vi "Actor Core.vi"(8 "Error In":errorcluster, 11 "CS++SeqEditor in":refnum<class "CS++SeqEditor.lvclass">) -> (0 "Error Out":errorcluster, 3 "Actor out":refnum<class "Actor.lvclass">)   [LabVIEW 2016, in "CS++SeqEditor.lvlib" / "CS++SeqEditor.lvclass"]
doc: "(<B>Filename</B>: Actor Framework.lvlib:Actor.lvclass:Actor Core.vi)\n\nReceives messages to the actor, reacts to them, and initiates any error handling that may shut the actor down.\n\nDescendant classes may override this VI to append parallel tasks for the actor to complete while it handles messages. Overrides use the Call Parent Method node."
uses:
  CS++SeqEditor.lvclass
  C:/User/Brand/LVP/CSPP-Dev/Packages/CSPP_Core/Actors/CS++BaseActor/CS++BaseActor.lvclass
  C:/User/Brand/LVP/CSPP-Dev/Packages/CSPP_Core/Actors/CS++GUIActor/CS++GUIActor.lvclass
  C:/Program Files (x86)/National Instruments/LabVIEW 2016/vi.lib/ActorFramework/Actor/Actor.lvclass
  <vilib>/ActorFramework/Actor/Actor.lvclass
  CSPP_Core/Libraries/Base/FGV Action.ctl
  CSPP_Core/Actors/CS++BaseActor/CS++BaseActor.lvclass/CS++BaseActor.ctl
  CSPP_Core/Actors/CS++GUIActor/CS++GUIActor.lvclass/CS++GUIActor.ctl
  CS++SeqEditor.lvclass/CS++SeqEditor.ctl
  <vilib>/ActorFramework/Actor/Actor.lvclass/Actor.ctl
  <vilib>/ActorFramework/Message Enqueuer/Message Enqueuer.lvclass/Message Enqueuer.ctl
  CS++SeqEditor Messages/Load Sequence Msg/Load Sequence Msg.lvclass/Load Sequence Msg.ctl
  CS++SeqEditor Messages/Save Sequence Msg/Save Sequence Msg.lvclass/Save Sequence Msg.ctl
  <vilib>/ActorFramework/Message/Message.lvclass
  CSPP_Core/Actors/CS++BaseActor/Read Object Name.vi
  CSPP_Core/Actors/CS++GUIActor/Read Associated Actor Name.vi
  CSPP_Core/Actors/CS++GUIActor/Read Stop-Event.vi
  CSPP_Core/Actors/CS++GUIActor/Read PV-Update.vi
  <vilib>/ActorFramework/Message Enqueuer/Init from Existing Queue.vi
  <vilib>/ActorFramework/Message Enqueuer/Enqueue.vi
  <vilib>/ActorFramework/Stop Msg/Stop Msg.lvclass
  C:/Program Files (x86)/National Instruments/LabVIEW 2016/vi.lib/ActorFramework/Message/Message.lvclass
  CS++SeqEditor Messages/Load Sequence Msg/Load Sequence Msg.lvclass
  CS++SeqEditor Messages/Save Sequence Msg/Save Sequence Msg.lvclass
  <vilib>/ActorFramework/Message Priority Queue/Priority Enqueue.vi
  CSPP_Core/Classes/CS++BaseClasses/Factory/CS++Factory.lvclass
  CSPP_Core/Classes/CS++ProcessVariables/ProcessVariable/PV.lvclass
  <vilib>/ActorFramework/Message Enqueuer/Message Enqueuer.lvclass
  CSPP_Core/Actors/CS++GUIActor/CS++GUIActor.lvclass
  CSPP_Core/Actors/CS++BaseActor/CS++BaseActor.lvclass
  CSPP_Core/Libraries/Base/CS++Base.lvlib
  CSPP_Core/Libraries/Utilities/CS++Utilities.lvlib
panel:
  out "Drop String":string
  in  "Message Tree":string(tree)
  out "Selected Path":path
  in  "Stop Button":bool
  out "Associated DeviceActor":string
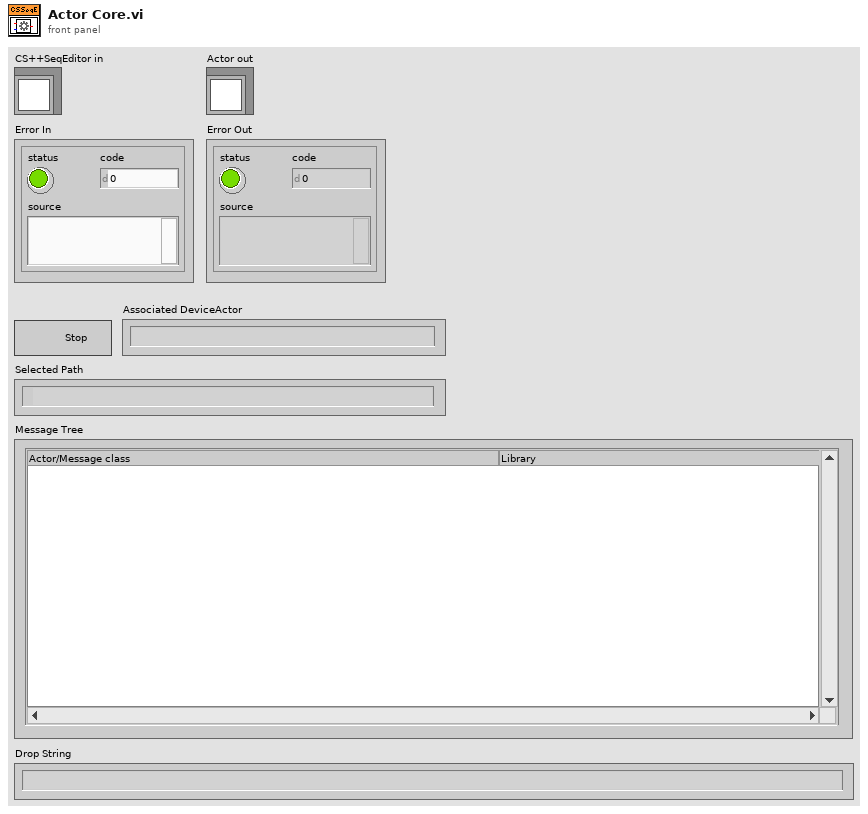
[diagram p1: front panel]
types:
  T1 = typedef "CS++Base.lvlib/FGV Action.ctl" = enum16{"add", "replace", "read", "remove", "reset", "get attributes"}
  T2 = enum32{"Invalid", "Standard", "Closed", "Hidden", "Minimized", "Maximized"}
  T3 = cluster{"Navigate Tree:Get Path":string[], "Actor Framework:Message":refnum<class "Message.lvclass">}
  T4 = typedef "LVMenuShortCut.ctl" = cluster{"include Shift key?":bool, "include Ctrl key?":bool, "shortcut key":string}
  T5 = cluster{"data name":string, "drag data":variant}[]
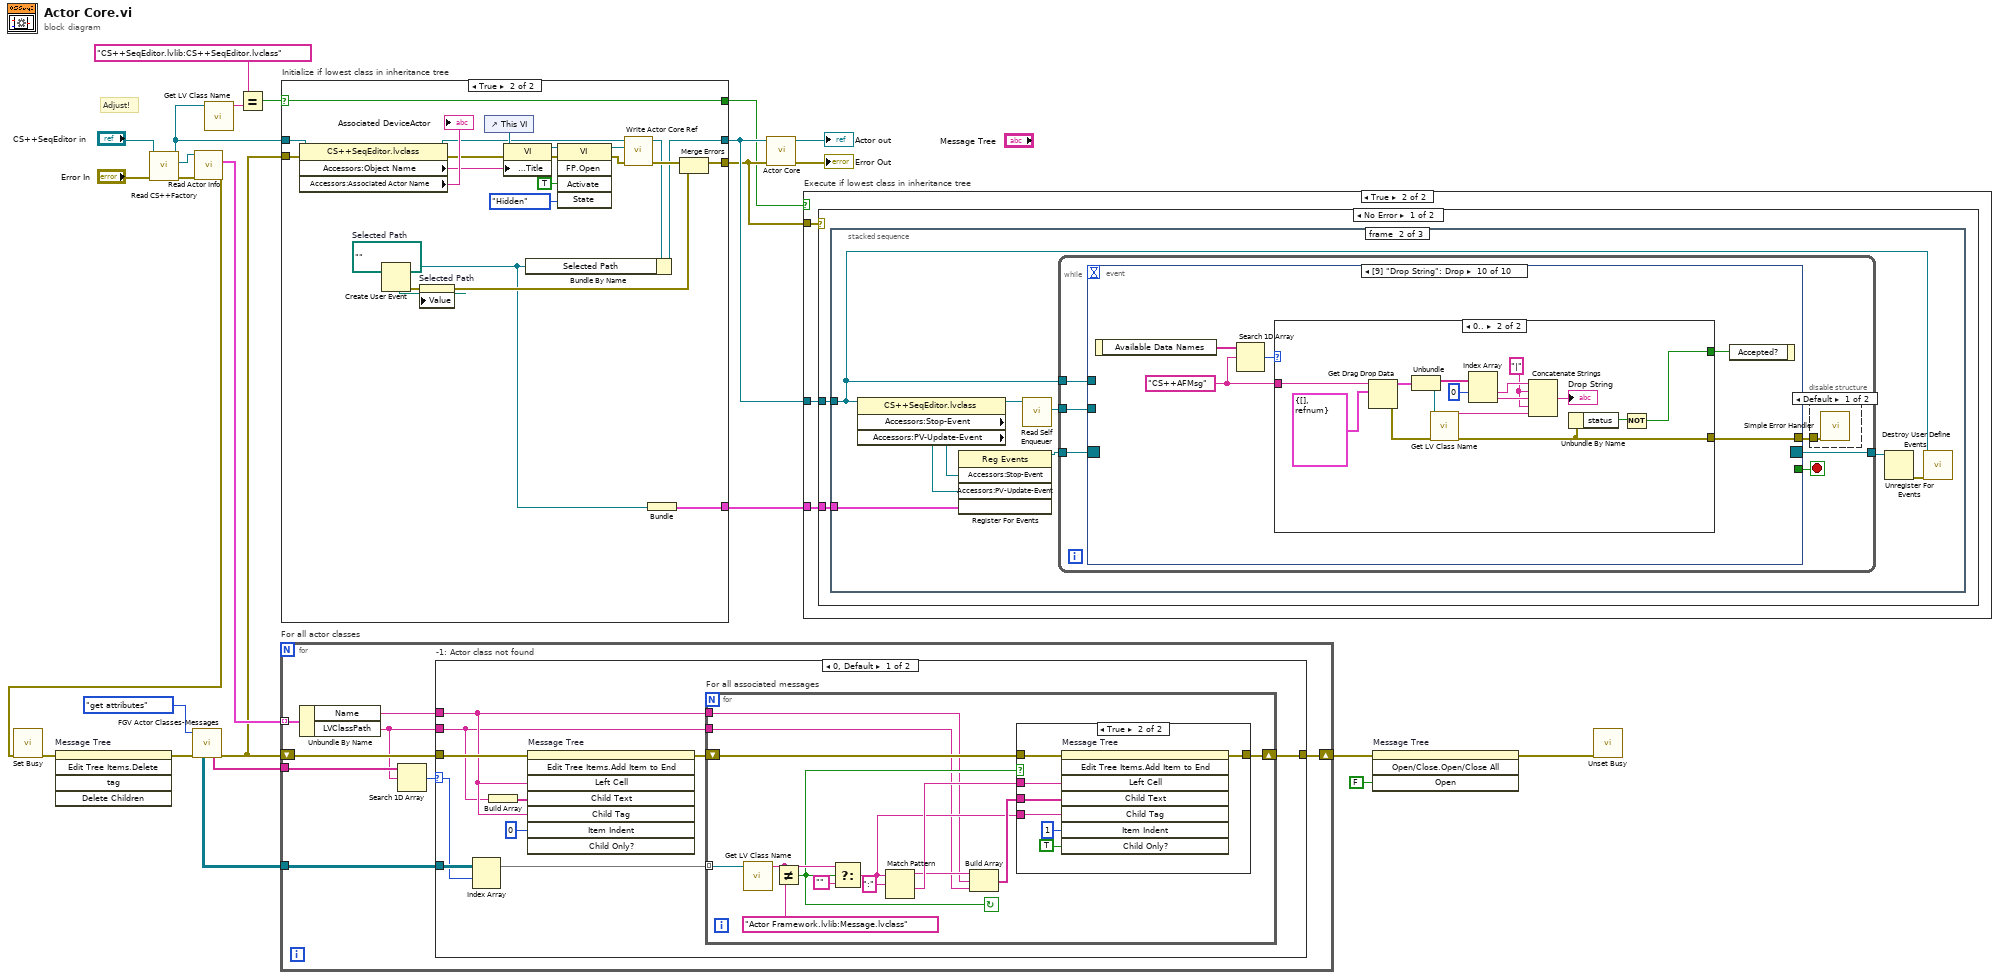
[diagram p0: block diagram]
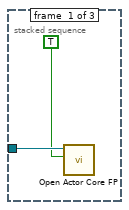
[diagram p5: hidden frame]
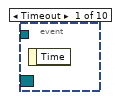
[diagram p6: hidden frame]
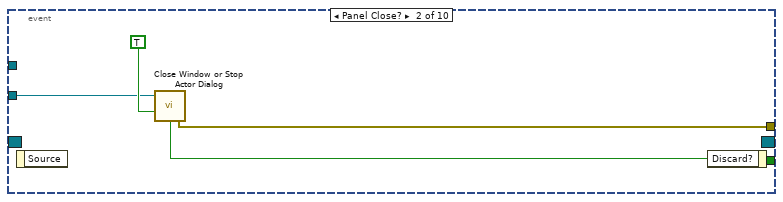
[diagram p7: hidden frame]
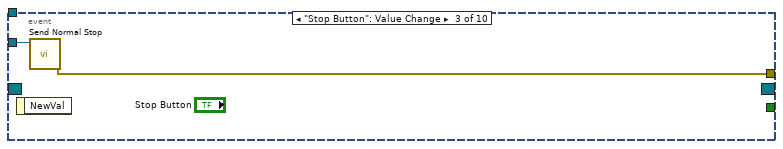
[diagram p8: hidden frame]
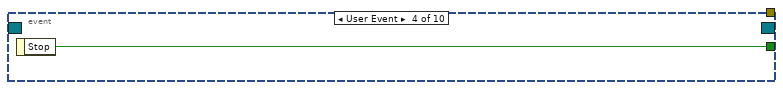
[diagram p9: hidden frame]
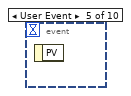
[diagram p10: hidden frame]
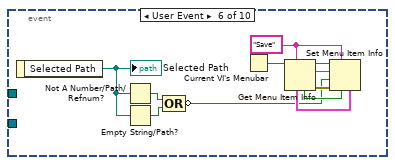
[diagram p11: hidden frame]
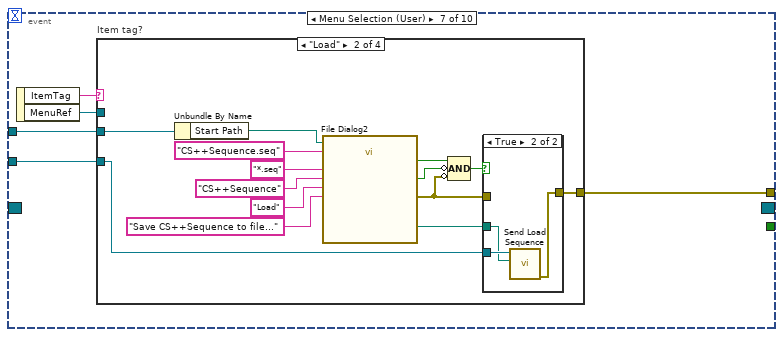
[diagram p12: hidden frame]
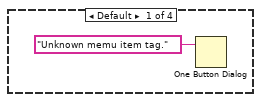
[diagram p13: hidden frame]
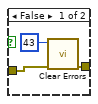
[diagram p14: hidden frame]
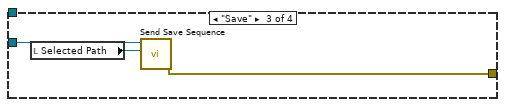
[diagram p15: hidden frame]
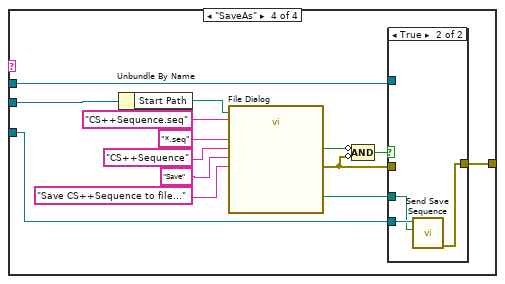
[diagram p16: hidden frame]
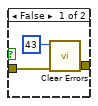
[diagram p17: hidden frame]
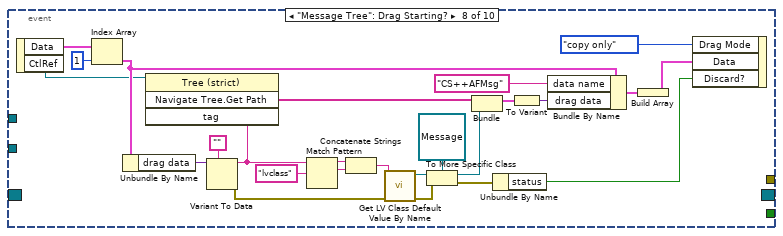
[diagram p18: hidden frame]
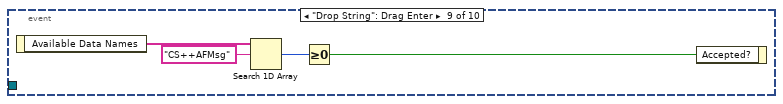
[diagram p19: hidden frame]
diagram:
  # "Adjust!"
  n1 = call "Read CS++Factory.vi"("error in (no error)"="Error In", "CS++BaseActor in"="CS++SeqEditor in") -> ("error out"=w7:errorcluster, "CS++Factory"=w8:refnum<class "CS++Factory.lvclass">, "CS++BaseActor out"=w4:refnum<class "CS++SeqEditor.lvclass">)  [unwired: 7 in]
  n2 = call-dynamic "Read Actor Info.vi"("Error In"=w7, "CS++Factory in"=w8) -> ("Error Out"=w2:errorcluster, "Actors"=w3:cluster{"Name":string, "LVClassPath":string}[])  [unwired: 7 in, 1 out]
  n3 = call <vilib>:"Set Busy.vi"("error in (no error)"=w2) -> ("error out"=w10:errorcluster)  [unwired: 9 in, 1 out]
  n4 = invoke on="Message Tree" class="Tree (strict)" method="Edit Tree Items.Delete"(error in=w10) -> (error out=w11:errorcluster)  [unwired: 4 in, 4 out]
  n5 = call "FGV Actor Classes-Messages.vi"("Error In"=w11, "Action (read)"=FGV_Action."get attributes") -> ("Error Out"=w1:errorcluster, "Class Names"=w14:string[], "CS++Messages"=w15:refnum<class "Message.lvclass">[][])  [unwired: 5 in, 2 out]
  n6 = call <vilib>:"Get LV Class Name.vi"("object"=w4) -> ("class name"=w25:string)  [unwired: 9 in, 1 out]
  n7 = Equal?(x="CS++SeqEditor.lvlib:CS++SeqEditor.lvclass" ("class name"), y=w25) -> (x = y?=w21:bool)
  n8 = for "For all actor classes" {
    tunnel: w15 -> [w33]
    tunnel: w14 -> [w28]
    shift-right: [w31] -> w12
    shift-left: w1 -> [w32]
    tunnel: w3 -> [w30] mode=indexing
    n9 = Unbundle By Name(w30) -> ("Name"=w29:string, "LVClassPath"=w27:string)
    n10 = Search 1D Array(1D array=w28, element=w27) -> (index of element=w26:i32)  [unwired: 1 in]
    n11 = case "-1: Actor class not found" shown="0, Default" w26 {
      selector: w26 -> [w36 _]
      tunnel: w33 -> [w43 _]
      tunnel: w32 -> [w42 w66]
      tunnel: [w39 w66] -> w31
      tunnel: w29 -> [w35 _]
      tunnel: w27 -> [w34 _]
      frame 0, Default {
        n12 = Index Array(array=w43, index (row)=w36) -> (element=w37:refnum<class "Message.lvclass">[])  [unwired: 1 in]
        n13 = Build Array(w34) -> (w38:string[])
        n14 = invoke on="Message Tree" class="Tree (strict)" method="Edit Tree Items.Add Item to End"(error in=w42, "Left Cell"=w35, "Child Text"=w38, "Child Tag"=w35, "Item Indent"=0 ("New Item Indentation")) -> (error out=w40:errorcluster)  [unwired: 3 in, 7 out]
        n15 = for "For all associated messages" {
          tunnel: w37 -> [w57] mode=indexing
          shift-right: [w51] -> w39
          shift-left: w40 -> [w52]
          tunnel: w35 -> [w45]
          tunnel: w34 -> [w44]
          stop <- w46 continue-if-true
          n16 = call <vilib>:"Get LV Class Name.vi"("object"=w57) -> ("class name"=w55:string)  [unwired: 9 in, 1 out]
          n17 = Not Equal?(x=w55, y="Actor Framework.lvlib:Message.lvclass") -> (x != y?=w46:bool)
          n18 = Select(t=w55, s=w46, f="") -> (s? t:f=w47:string)
          n19 = Match Pattern(string=w47, regular expression=":") -> (before substring=w49:string, after substring=w50:string)  [unwired: 1 in, 2 out]
          n20 = Build Array(w49, w45, w44) -> (w48:string[])
          n21 = case shown="True" w46 {
            tunnel: w52 -> [w58 w65]
            tunnel: [w58 w64] -> w51
            tunnel: w50 -> [_ w63]
            tunnel: w48 -> [_ w62]
            tunnel: w47 -> [_ w61]
            frame False {
            }
            frame True {
              n22 = invoke on="Message Tree" class="Tree (strict)" method="Edit Tree Items.Add Item to End"(error in=w65, "Left Cell"=w63, "Child Text"=w62, "Child Tag"=w61, "Item Indent"=1 ("New Item Indentation"), "Child Only?"=TRUE) -> (error out=w64:errorcluster)  [unwired: 2 in, 7 out]
            }
          }
        }
      }
      frame -1 {
      }
    }
  }
  n23 = case "Initialize if lowest class in inheritance tree" shown="True" w21 {
    selector: w21 -> [w69 w90]
    tunnel: w1 -> [w67 w87]
    tunnel: w4 -> [w68 w88]
    tunnel: [w68 w75] -> w23
    tunnel: [w67 w73] -> w22
    tunnel: [w69 w90] -> w20
    tunnel: [_ w70] -> w17
    frame False {
    }
    frame True {
      w77 = path ""  # Selected Path
      n24 = property class="CS++SeqEditor.lvclass"(reference=w88, error in=w87) -> (reference out=w78:refnum<class "CS++SeqEditor.lvclass">, error out=w80:errorcluster, "Accessors:Object Name"=w79:string, "Accessors:Associated Actor Name"=→"Associated DeviceActor":string)
      n25 = Create User Event(user event datatype=w77) -> (user event=w71:refnum<user-event>, error out=w74:errorcluster)  [unwired: 1 in]
      n26 = property on="Selected Path" class="Path"(error in=w74, "Value"=w77) -> (error out=w72:errorcluster)  [unwired: 1 in, 1 out]
      n27 = control-ref of="This VI"() -> (w83:refnum<vi>)
      n28 = property class="VI"(reference=w83, error in=w80, "Front Panel.Title"=w79) -> (reference out=w82:refnum<vi>, error out=w81:errorcluster)
      n29 = invoke class="VI" method="FP.Open"(reference=w82, error in=w81, "Activate"=TRUE ("Activate?"), "State"=T2."Hidden") -> (reference out=w89:refnum<vi>, error out=w85:errorcluster)  [unwired: 1 in, 3 out]
      n30 = call "Write Actor Core Ref.vi"("error in (no error)"=w85, "Actor Core Ref"=w89, "CS++BaseActor in"=w78) -> ("error out"=w84:errorcluster, "CS++BaseActor out"=w76:refnum<class "CS++SeqEditor.lvclass">)  [unwired: 7 in]
      n31 = Bundle By Name(cluster=w76, "Selected Path"=w71) -> (w75:refnum<class "CS++SeqEditor.lvclass">)
      n32 = Bundle("Selected Path"=w71) -> (w70:cluster{"Selected Path":refnum<user-event>})  [unwired: 1 in]
      n33 = Merge Errors(w84, w72) -> (w73:errorcluster)
    }
  }
  n34 = call-parent "Actor Core.vi"("error in"=w22, "CS++GUIActor in"=w23) -> ("error out"=→"Error Out":errorcluster, "Actor out"=→"Actor out":refnum<class "Actor.lvclass">)  [unwired: 8 in]
  n35 = case "Execute if lowest class in inheritance tree" shown="True" w20 {
    tunnel: w23 -> [_ w95]
    tunnel: w22 -> [_ w94]
    tunnel: w17 -> [_ w93]
    frame False {
    }
    frame True {
      n36 = case shown="No Error" w94 {
        tunnel: w95 -> [w97 _]
        tunnel: w93 -> [w96 _]
        frame No Error {
          n37 = stacked-sequence {
            tunnel: w97 -> [w99 w101 w232]
            tunnel: w96 -> [_ w100 _]
            frame #0 {
              n38 = call "Open Actor Core FP.vi"("Open FP (F)"=TRUE, "CS++BaseActor in"=w99) -> ()  [unwired: 8 in, 2 out]
            }
            frame #1 {
              n39 = property class="CS++SeqEditor.lvclass"(reference=w101) -> (reference out=w106:refnum<class "CS++SeqEditor.lvclass">, "Accessors:Stop-Event"=w103:refnum<user-event>, "Accessors:PV-Update-Event"=w102:refnum<user-event>)  [unwired: 1 in, 1 out]
              n40 = register-events(w103, w102, w100) -> (reference out=w104:refnum<event-registration>)  [unwired: 2 in, 1 out]
              n41 = call <vilib>:"Read Self Enqueuer.vi"("Actor"=w106) -> ("Self Enqueuer"=w105:refnum<class "Message Enqueuer.lvclass">)  [unwired: 10 in]
              n42 = while {
                tunnel: w104 -> [w114]
                tunnel: [w112] -> w108
                tunnel: w105 -> [w110]
                tunnel: w101 -> [w109]
                stop <- w113 stop-if-true
                n43 = event shown="[9] \"Drop String\": Drop" {
                  selector: w114 -> [_ _ _ _ _ _ _ _ _ _]
                  dyn-events: [_ _ _ _ _ _ _ _ _ _] -> w112
                  timeout: _ -> [_ _ _ _ _ _ _ _ _ _]
                  tunnel: [_ _ _ w120 _ _ _ _ _ _] -> w113
                  tunnel: [_ w115 w119 _ _ _ w132 _ _ w211] -> w111
                  tunnel: w110 -> [_ w116 w118 _ _ _ w133 _ _ _]
                  tunnel: w109 -> [_ _ _ _ _ _ w135 _ _ _]
                  event Timeout {
                    n44 = event-data() -> ()  [unwired: 1 in, 1 out]
                  }
                  event Panel Close? {
                    n45 = event-data() -> ()  [unwired: 1 in, 1 out]
                    n46 = call "Close Window or Stop Actor Dialog.vi"("Self Enqueuer"=w116) -> ("Error Out"=w115:errorcluster)  [unwired: 2 in]
                    n47 = event-data("Discard?"=TRUE) -> ()  [unwired: 1 in, 1 out]
                  }
                  event "Stop Button": Value Change {
                    n48 = event-data() -> ()  [unwired: 1 in, 1 out]
                    n49 = call <vilib>:"Send Normal Stop.vi"("Message Enqueuer"=w118) -> ("error out"=w119:errorcluster)  [unwired: 10 in]
                  }
                  event User Event {
                    n50 = event-data() -> ("Stop"=w120:bool)  [unwired: 1 in]
                  }
                  event User Event {
                    n51 = event-data() -> ()  [unwired: 1 in, 1 out]
                  }
                  event User Event {
                    w128 = "Save"
                    n52 = event-data() -> ("Selected Path"=w126:path)  [unwired: 1 in]
                    "Selected Path" <- w126
                    n53 = Not A Number/Path/Refnum?(number/path/refnum=w126) -> (NaN/Path/Refnum?=w125:bool)
                    n54 = Empty String/Path?(string/path=w126) -> (empty?=w124:bool)
                    n55 = Compound Arithmetic op=OR(w125, w124) -> (invert w121:bool)
                    n56 = Current VI's Menubar() -> (w123:refnum<k9>)
                    n57 = Get Menu Item Info(7:w128, 11:w123) -> (0:w131:errorcluster, 2:w130:string, 3:w129:refnum<k9>, 4:w122:bool, 6:w127:T4)  [unwired: 1 in, 2 out]
                    n58 = Set Menu Item Info(4:w127, 6:w122, 7:w128, 8:w131, 9:w121, 10:w130, 11:w129) -> ()  [unwired: 2 out]
                  }
                  event Menu Selection (User) {
                    n59 = event-data() -> ("ItemTag"=w136:string, "MenuRef"=w134:refnum<k9>)  [unwired: 1 in]
                    n60 = case "Item tag?" shown="\"Load\"" w136 {
                      tunnel: w135 -> [_ w146 _ w169]
                      tunnel: w134 -> [_ _ _ w166]
                      tunnel: w133 -> [_ w141 w160 w164]
                      tunnel: [_ w139 w158 w162] -> w132
                      frame Default {
                        n61 = One Button Dialog(message="Unknown memu item tag.") -> ()  [unwired: 1 in, 1 out]
                      }
                      frame "Load" {
                        n62 = Unbundle By Name(w146) -> ("Start Path"=w145:path)
                        n63 = call "File Dialog2"("start path"=w145, "prompt"="Save CS++Sequence to file...", "button label"="Load", "default name"="CS++Sequence.seq", "pattern (all files)"="*.seq", "pattern label"="CS++Sequence") -> ("selected path"=w140:path, "exists"=w144:bool, "cancelled"=w143:bool, "error out"=w138:errorcluster)  [unwired: 6 in]
                        n64 = Compound Arithmetic op=AND(w144, invert w143, invert w138) -> (w142:bool)
                        n65 = case shown="True" w142 {
                          tunnel: w141 -> [_ w157]
                          tunnel: w140 -> [_ w156]
                          tunnel: [w153 w155] -> w139
                          tunnel: w138 -> [w154 _]
                          frame False {
                            n66 = call <vilib>:"Clear Errors.vi"("error in (no error)"=w154, "specific error code to clear (0: all)"=43) -> ("error out"=w153:errorcluster)  [unwired: 4 in, 1 out]
                          }
                          frame True {
                            n67 = call "Send Load Sequence.vi"("Selected Path"=w156, "Message Enqueuer"=w157) -> ("error out"=w155:errorcluster)  [unwired: 8 in, 1 out]
                          }
                        }
                      }
                      frame "Save" {
                        n68 = local read "Selected Path"() -> (w159:path)
                        n69 = call "Send Save Sequence.vi"("Selected Path"=w159, "Message Enqueuer"=w160) -> ("error out"=w158:errorcluster)  [unwired: 8 in, 1 out]
                      }
                      frame "SaveAs" {
                        n70 = Unbundle By Name(w169) -> ("Start Path"=w168:path)
                        n71 = call "File Dialog"("start path"=w168, "prompt"="Save CS++Sequence to file...", "button label"="Save", "default name"="CS++Sequence.seq", "pattern (all files)"="*.seq", "pattern label"="CS++Sequence") -> ("selected path"=w163:path, "cancelled"=w165:bool, "error out"=w161:errorcluster)  [unwired: 6 in, 1 out]
                        n72 = Compound Arithmetic op=AND(invert w165, invert w161) -> (w167:bool)
                        n73 = case shown="True" w167 {
                          tunnel: w166 -> [_ _]
                          tunnel: w164 -> [_ w180]
                          tunnel: w163 -> [_ w179]
                          tunnel: [w176 w178] -> w162
                          tunnel: w161 -> [w177 _]
                          frame False {
                            n74 = call <vilib>:"Clear Errors.vi"("error in (no error)"=w177, "specific error code to clear (0: all)"=43) -> ("error out"=w176:errorcluster)  [unwired: 4 in, 1 out]
                          }
                          frame True {
                            n75 = call "Send Save Sequence.vi"("Selected Path"=w179, "Message Enqueuer"=w180) -> ("error out"=w178:errorcluster)  [unwired: 8 in, 1 out]
                          }
                        }
                      }
                    }
                  }
                  event "Message Tree": Drag Starting? {
                    n76 = event-data() -> ("Data"=w193:T5, "CtlRef"=w184:refnum<vi>)  [unwired: 1 in]
                    n77 = Index Array(array=w193, index=1) -> (element=w204:cluster{"data name":string, "drag data":variant})
                    n78 = Unbundle By Name(w204) -> ("drag data"=w202:variant)
                    n79 = Variant To Data(type="", Variant=w202) -> (data=w185:string, error out=w188:errorcluster)  [unwired: 1 in]
                    n80 = invoke class="Tree (strict)" method="Navigate Tree.Get Path"(reference=w184, "tag"=w185) -> ("Navigate Tree:Get Path"=w183:string[])  [unwired: 2 in, 3 out]
                    n81 = Match Pattern(string=w185, regular expression="lvclass") -> (before substring=w196:string, match substring=w195:string)  [unwired: 1 in, 2 out]
                    n82 = Concatenate Strings(w196, w195) -> (w189:string)
                    n83 = call <vilib>:"Get LV Class Default Value By Name.vi"("error in (no error)"=w188, "class name"=w189) -> ("error out"=w191:errorcluster, "object"=w192:refnum<class>)  [unwired: 8 in]
                    n84 = To More Specific Class(target class=refnum<class "Message.lvclass"> refnum ("Actor Framework:Message"), reference=w192, error in=w191) -> (specific class reference=w182:refnum<class "Message.lvclass">, error out=w186:errorcluster)
                    n85 = Bundle("Navigate Tree:Get Path"=w183, "Actor Framework:Message"=w182) -> (w181:T3)  [unwired: 1 in]
                    n86 = Unbundle By Name(w186) -> ("status"=w187:bool)
                    n87 = To Variant(anything=w181) -> (Variant=w194:variant)
                    n88 = Bundle By Name(cluster=w204, "data name"="CS++AFMsg", "drag data"=w194) -> (w199:cluster{"data name":string, "drag data":variant})
                    n89 = Build Array(w199) -> (w198:T5)
                    n90 = event-data("Drag Mode"=enum32{"copy or move", "copy only", "move only"}."copy only", "Data"=w198, "Discard?"=w187) -> ()  [unwired: 1 in, 1 out]
                  }
                  event "Drop String": Drag Enter {
                    n91 = event-data() -> ("Available Data Names"=w208:string[])  [unwired: 1 in]
                    n92 = Search 1D Array(1D array=w208, element="CS++AFMsg" ("data name")) -> (index of element=w209:i32)  [unwired: 1 in]
                    n93 = Greater Or Equal To 0?(x=w209) -> (x >= 0?=w206:bool)
                    n94 = event-data("Accepted?"=w206) -> ()  [unwired: 1 in, 1 out]
                  }
                  event "Drop String": Drop {
                    w213 = "CS++AFMsg" ("data name")
                    n95 = event-data() -> ("Available Data Names"=w214:string[])  [unwired: 1 in]
                    n96 = Search 1D Array(1D array=w214, element=w213) -> (index of element=w212:i32)  [unwired: 1 in]
                    n97 = case shown="0.." w212 {
                      tunnel: w213 -> [_ w227]
                      tunnel: [_ w217] -> w211
                      tunnel: [_ w215] -> w210
                      frame Default {
                      }
                      frame 0.. {
                        w219 = "|"
                        n98 = Get Drag Drop Data(8:T3 {"Navigate Tree:Get Path"=[], "Actor Framework:Message"=refnum} ("output cluster"), 9:w227) -> (0:w228:errorcluster, 3:w229:T3)  [unwired: 1 in]
                        n99 = Unbundle(w229) -> ("Navigate Tree:Get Path"=w224:string[], "Actor Framework:Message"=w225:refnum<class "Message.lvclass">)
                        n100 = call <vilib>:"Get LV Class Name.vi"("error in (no error)"=w228, "object"=w225) -> ("error out"=w217:errorcluster, "class name"=w220:string)  [unwired: 8 in]
                        n101 = Index Array(array=w224, index #1=0 ("index")) -> (element #1=w222:string, element #2=w221:string)  [unwired: 1 in]
                        n102 = Concatenate Strings(w222, w219, w221, w219, w220) -> (→"Drop String":string)
                        n103 = Unbundle By Name(w217) -> ("status"=w216:bool)
                        n104 = Not(x=w216) -> (.not. x?=w215:bool)
                      }
                    }
                    n105 = event-data("Accepted?"=w210) -> ()  [unwired: 1 in, 1 out]
                  }
                }
                n106 = disable-structure shown="Default" {
                  disable-tunnel: w111 -> [w230 _]
                  frame condition #0 (active) {
                    n107 = call <vilib>:"Simple Error Handler.vi"("error in (no error)"=w230) -> ()  [unwired: 4 in, 5 out]
                  }
                  frame condition #1 {
                  }
                }
              }
              n108 = Unregister For Events(event registration refnum=w108) -> (error out=w107:errorcluster)  [unwired: 1 in]
              n109 = call-dynamic "Destroy User Define Events.vi"("error in (no error)"=w107, "CS++SeqEditor in"=w101) -> ()  [unwired: 8 in, 2 out]
            }
            frame #2 {
              n110 = call "Open Actor Core FP.vi"("Open FP (F)"=FALSE, "CS++BaseActor in"=w232) -> ()  [unwired: 8 in, 2 out]
            }
          }
        }
        frame Error {
        }
      }
    }
  }
  n111 = invoke on="Message Tree" class="Tree (strict)" method="Open/Close.Open/Close All"(error in=w12, "Open"=FALSE ("Open?")) -> (error out=w9:errorcluster)  [unwired: 2 in, 3 out]
  n112 = call <vilib>:"Unset Busy.vi"("error in (no error)"=w9) -> ()  [unwired: 10 in, 1 out]
